vi "Set Tester Tx.vi"(8 "error in (no error)":errorcluster, 10 "Auto/Manual":bool=TRUE, 11 "Panel in":refnum<class "Panel.lvclass">) -> (0 "error out":errorcluster, 3 "Panel out":refnum<class "Panel.lvclass">)   [LabVIEW 2021, in "Panel.lvlib" / "Panel.lvclass"]
uses:
  Panel.lvclass
  Panel.lvclass/Panel.ctl
  <vilib>/OPCUA/server/Read Variant.vi
  <vilib>/OPCUA/NI OPC UA Server.lvlib
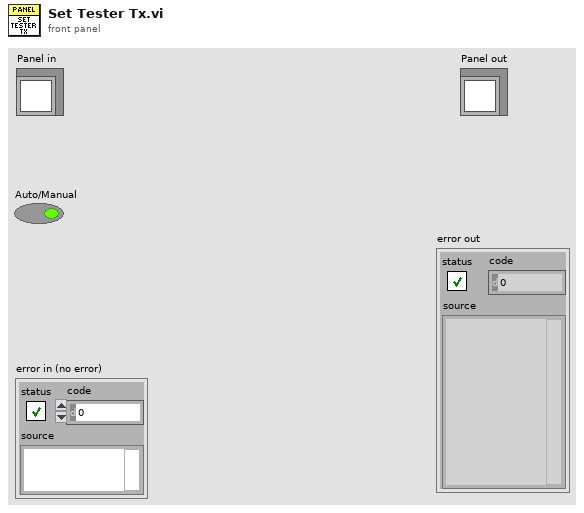
[diagram p1: front panel]
types:
  T1 = typedef "OPC UA Server Refnum.ctl" = refnum<k21>
  T2 = typedef "Panel.lvlib/Panel.lvclass/Tester Rx Dataset.ctl" = cluster{"Start":bool, "NestStatus":bool, "PalletID":u32, "BarcodeData":string, "StepEcho":u32, "Cylinder_1":bool, "Cylinder_2":bool, "Cylinder_3":bool, "Cylinder_4":bool, "Cylinder_5":bool, "ResultsAck":bool, "Reset":bool, "Stop":bool, "FaultCode":u32}
  T3 = typedef "Panel.lvlib/Panel.lvclass/Tester Tx Dataset.ctl" = cluster{"Fault":bool, "StepNo":u32, "Ready":bool, "HighVoltage":bool, "TestRunning":bool, "ResultsReady":bool, "Results":u32, "ElapsedTime":u32, "Online":bool, "TimeCompleted":i32[], "Timeout":bool}
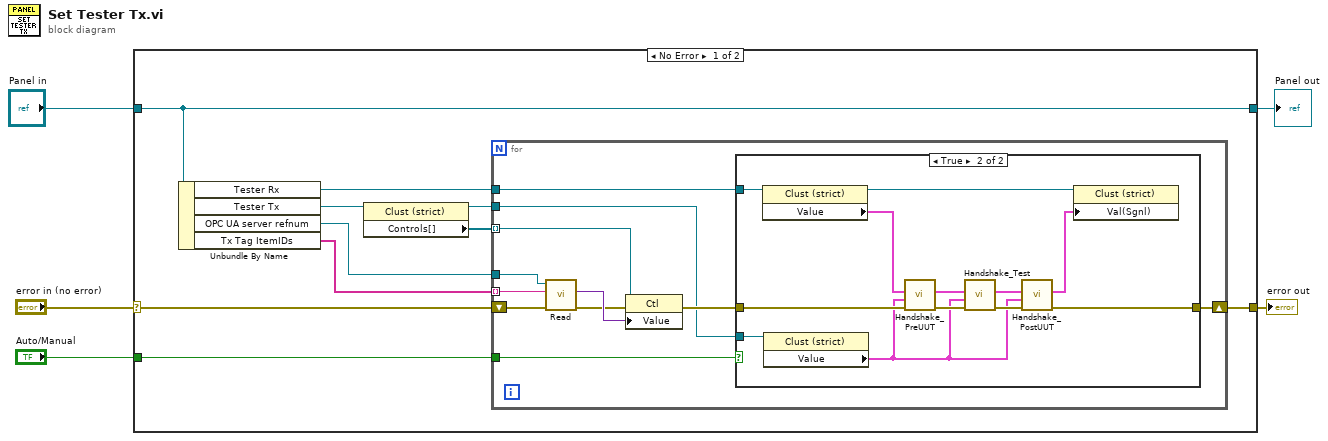
[diagram p0: block diagram]
diagram:
  n1 = case shown="No Error" "error in (no error)" {
    selector: "error in (no error)" -> [w10 w41]
    tunnel: [w9 w41] -> w4
    tunnel: [w11 w40] -> w2
    tunnel: "Panel in" -> [w11 w40]
    tunnel: "Auto/Manual" -> [w8 _]
    frame No Error {
      n2 = Unbundle By Name(w11) -> ("Tester Rx"=w6:refnum<vi>, "Tester Tx"=w12:refnum<vi>, "OPC UA server refnum"=w14:T1, "Tx Tag ItemIDs"=w15:string[])
      n3 = property class="Clust (strict)"(reference=w12) -> (reference out=w7:refnum<vi>, "Controls[]"=w13:refnum<vi>[])  [unwired: 1 in, 1 out]
      n4 = for {
        tunnel: w14 -> [w26]
        tunnel: w15 -> [w24] mode=indexing
        shift-right: [w18] -> w9
        shift-left: w10 -> [w25]
        tunnel: w13 -> [w23] mode=indexing
        tunnel: w8 -> [w20]
        tunnel: w7 -> [w17]
        tunnel: w6 -> [w16]
        n5 = call-poly <vilib>:"Read.vi"("error in (no error)"=w25, "node ID"=w24, "OPC UA server refnum in"=w26) -> ("error out"=w21:errorcluster, "value"=w22:variant)  [unwired: 4 in, 3 out]
        n6 = property class="Ctl"(reference=w23, error in=w21, "Value"=w22) -> (error out=w19:errorcluster)  [unwired: 1 out]
        n7 = case shown="True" w20 {
          tunnel: w19 -> [w27 w39]
          tunnel: [w27 w36] -> w18
          tunnel: w17 -> [_ w35]
          tunnel: w16 -> [_ w28]
          frame False {
          }
          frame True {
            n8 = property class="Clust (strict)"(reference=w28) -> (reference out=w30:refnum<vi>, "Value"=w33:T2)  [unwired: 1 in, 1 out]
            n9 = property class="Clust (strict)"(reference=w35) -> ("Value"=w34:T3)  [unwired: 1 in, 2 out]
            n10 = call "Handshake_PreUUT.vi"("error in"=w39, "Tester Tx"=w34, "Tester Rx In"=w33) -> ("error out"=w38:errorcluster, "Tester Rx out"=w29:T2)  [unwired: 7 in]
            n11 = call "Handshake_Test.vi"("error in"=w38, "Tester Tx"=w34, "Tester Rx In"=w29) -> ("error out"=w37:errorcluster, "Tester Rx out"=w32:T2)  [unwired: 7 in]
            n12 = call "Handshake_PostUUT.vi"("error in"=w37, "Tester Tx"=w34, "Tester Rx In"=w32) -> ("error out"=w36:errorcluster, "Tester Rx out"=w31:T2)  [unwired: 7 in]
            n13 = property class="Clust (strict)"(reference=w30, "Val(Sgnl)"=w31) -> ()  [unwired: 1 in, 2 out]
          }
        }
      }
    }
    frame Error {
    }
  }
  "error out" <- w4
  "Panel out" <- w2
